vi "update_params.vi"(0 "W1 in":dbl[][](array[numeric]), 1 "dW1":dbl[][](array[numeric]), 2 "db1":dbl[](array[numeric]), 5 "b1 in":dbl[](array[numeric]), 7 "W2 in":dbl[][](array[numeric]), 9 "b2 in":dbl[](array[numeric]), 11 "alpha":dbl, 12 "dW2":dbl[][](array[numeric]), 13 "db2":dbl[](array[numeric])) -> (4 "W1 out":dbl[][](array[numeric]), 6 "b1 out":dbl[](array[numeric]), 8 "W2 out":dbl[][](array[numeric]), 10 "b2 out":dbl[](array[numeric]))   [LabVIEW 2023]
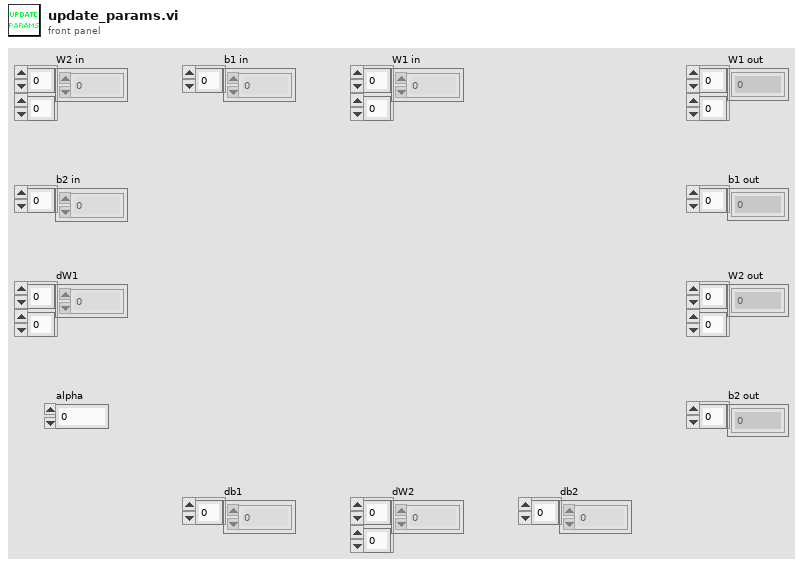
[diagram p1: front panel]
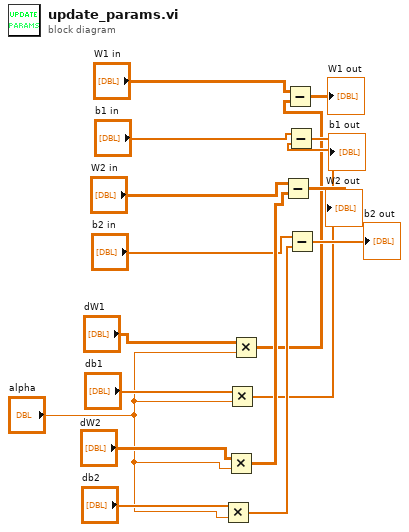
[diagram p0: block diagram]
diagram:
  n1 = Multiply(x="db2", y="alpha") -> (x*y=w13:dbl[])
  n2 = Multiply(x="dW2", y="alpha") -> (x*y=w12:dbl[][])
  n3 = Multiply(x="db1", y="alpha") -> (x*y=w11:dbl[])
  n4 = Multiply(x="dW1", y="alpha") -> (x*y=w10:dbl[][])
  n5 = Subtract(x="W2 in", y=w12) -> (x-y=→"W2 out":dbl[][])
  n6 = Subtract(x="W1 in", y=w10) -> (x-y=→"W1 out":dbl[][])
  n7 = Subtract(x="b1 in", y=w11) -> (x-y=→"b1 out":dbl[])
  n8 = Subtract(x="b2 in", y=w13) -> (x-y=→"b2 out":dbl[])
